vi "Relative2AbsoluteCords.vi"(2 "Obj bearing":dbl, 3 "Obj distance":dbl, 4 "Robot":cluster{"X":dbl, "Y":dbl, "Bearing":dbl}) -> (0 "Obj Y-cord":dbl, 1 "Obj X-cord":dbl)   [LabVIEW 2009]
doc: "Relative cords from camera to absolute cordinates in the virtual map"
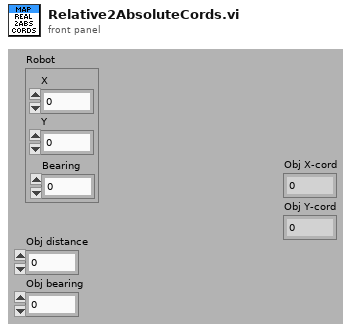
[diagram p1: front panel]
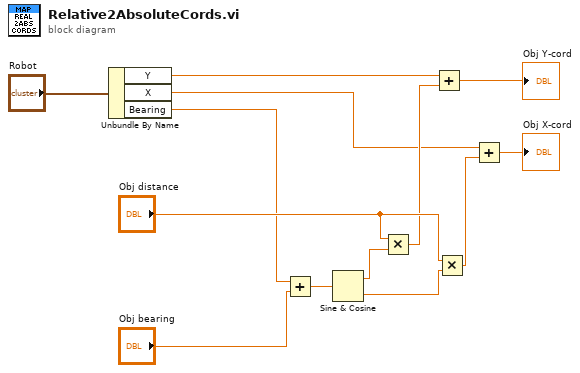
[diagram p0: block diagram]
diagram:
  n1 = Unbundle By Name("Robot") -> ("Y"=w3:dbl, "X"=w2:dbl, "Bearing"=w1:dbl)
  n2 = Add(x=w1, y="Obj bearing") -> (x+y=w12:dbl)
  n3 = Sine & Cosine(0:w12) -> (1:w9:dbl, 2:w11:dbl)
  n4 = Multiply(x="Obj distance", y=w9) -> (x*y=w5:dbl)
  n5 = Add(x=w3, y=w5) -> (x+y=→"Obj Y-cord":dbl)
  n6 = Multiply(x="Obj distance", y=w11) -> (x*y=w8:dbl)
  n7 = Add(x=w2, y=w8) -> (x+y=→"Obj X-cord":dbl)
